vi "initial-Pos-XY.vi"(8 "error in (no error)":errorcluster) -> (0 "error out":errorcluster, 2 "Y position":dbl, 3 "X position":dbl)   [LabVIEW 2014]
doc: "André Romero - 2023\nandretec@ifsc.usp.br\nIFSC - USP"
uses:
  Global Motors.vi
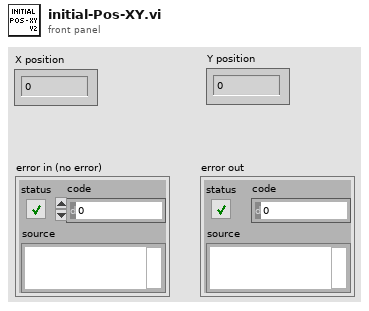
[diagram p1: front panel]
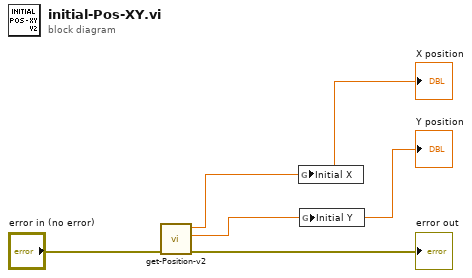
[diagram p0: block diagram]
diagram:
  n1 = call "get-Position-v2.vi"("error in (no error)"="error in (no error)") -> ("error out"=→"error out":errorcluster, "Position Y"=w1:dbl, "Position X"=w2:dbl)  [unwired: 7 in, 1 out]
  "X position" <- w2
  "Y position" <- w1
  n2 = global write "Global Motors.vi" "Initial X"(w2) -> ()
  n3 = global write "Global Motors.vi" "Initial Y"(w1) -> ()
